vi "RSZVB Set Logical Port Common Ref Impedance.vi"(6 "Real (25 Ohm)":dbl=25.0 format="%^.3e", 7 "Imaginary (0 Ohm)":dbl format="%^.3e", 8 "error in (no error)":errorcluster {"code" format="%.0x"}, 9 "Port (1)":i32=1, 10 "Channel (1)":i32=1, 11 "VISA session":refnum<visa-resource-name>) -> (0 "error out":errorcluster {"code" format="%.0x"}, 3 "dup VISA session":refnum<visa-resource-name>)   [LabVIEW 2011]
doc: "This VI specifies the complex common mode reference impedance for the balanced (logical) port numbered <log_port>. \n\nRemote-control command(s):\n[SENSe<Ch>:]LPORt<log_port>:ZCOMmon <real>[, <imaginary>]"
uses:
  _utility/RSZVB Global Data.vi
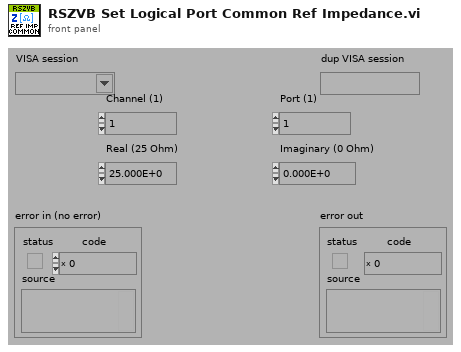
[diagram p1: front panel]
types:
  T1 = cluster{"Error Checking (T: On)":bool, "Installed Options":string[], "Data Valid?":bool, "Ports":i32, "Model":string[], "Option Checking (T: On)":bool}[]
  T2 = cluster{"Error Checking (T: On)":bool, "Installed Options":string[], "Data Valid?":bool, "Ports":i32, "Model":string[], "Option Checking (T: On)":bool}
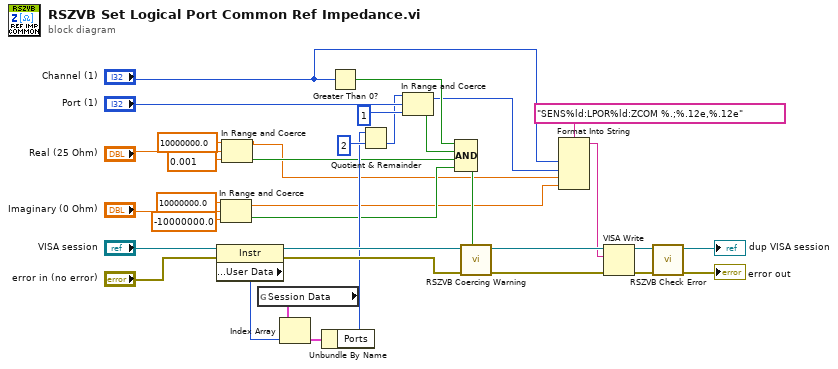
[diagram p0: block diagram]
diagram:
  n1 = property class="Instr"(reference="VISA session", error in="error in (no error)") -> (reference out=w34:refnum<visa-resource-name>, error out=w33:errorcluster, "General Settings:User Data"=w32:u32)
  n2 = In Range and Coerce(upper limit=10000000.0 ("lower limit"), x="Imaginary (0 Ohm)", lower limit=-10000000.0) -> (coerced(x)=w1:dbl, In Range?=w13:bool)
  n3 = In Range and Coerce(upper limit=10000000.0 ("lower limit"), x="Real (25 Ohm)", lower limit=0.001) -> (coerced(x)=w2:dbl, In Range?=w14:bool)
  n4 = global read "RSZVB Global Data.vi" "Session Data"() -> (w31:T1)
  n5 = Index Array(array=w31, index=w32) -> (element=w30:T2)
  n6 = Unbundle By Name(w30) -> ("Ports"=w21:i32)
  n7 = Greater Than 0?(x="Channel (1)") -> (x > 0?=w29:bool)
  n8 = Quotient & Remainder(x=w21, y=2) -> (floor(x/y)=w16:i32)  [unwired: 1 out]
  n9 = In Range and Coerce(upper limit=w16, x="Port (1)", lower limit=1) -> (coerced(x)=w3:i32, In Range?=w15:bool)
  n10 = Compound Arithmetic op=AND(w29, w15, w14, w13) -> (w28:bool)
  n11 = call "RSZVB Coercing Warning.vi"("In Range?"=w28, "error in (no error)"=w33, "VISA session"=w34) -> ("error out"=w8:errorcluster, "dup VISA session"=w7:refnum<visa-resource-name>)  [unwired: 7 in]
  n12 = Format Into String(format string="SENS%ld:LPOR%ld:ZCOM %.;%.12e,%.12e", "Channel (1)", w3, w2, w1) -> (resulting string=w6:string)  [unwired: 2 in, 1 out]
  n13 = VISA Write(VISA resource name=w7, write buffer=w6, error in (no error)=w8) -> (VISA resource name out=w12:refnum<visa-resource-name>, error out=w11:errorcluster)  [unwired: 1 out]
  n14 = call "RSZVB Check Error.vi"("error in (no error)"=w11, "VISA session"=w12) -> ("error out"=→"error out":errorcluster, "dup VISA session"=→"dup VISA session":refnum<visa-resource-name>)  [unwired: 8 in]
